vi "OCT with Classes - ATS6350.vi"() -> ()   [LabVIEW 2014]
doc: "I. Description:\nThis example demonstrates how to acquire a continuous amount of data (Waveform) using the DAQ device's internal clock.\n\nII. Instructions for Running:\n1. Create an analog input voltage channel.\n2. Set the rate for the sample clock. Additionally, define the sample mode to be continuous.\n3. Call the Start VI to start the acquisition.\n4. Read the waveform data in a loop until the user hits the stop button or an error occurs.\nNote: This example reads data from one or more channels and returns an array of data. Use the Index Array function to access an individual channel of data.\n5. Call the Clear Task VI to clear the Task.\n6. Use the popup dialog box to display an error if any.\n\nIV. I/O Connections Overview:\nMake sure your signal input terminal matches the Physical Channel I/O Control. For further connection information, refer to your hardware reference manual."
uses:
  Type Defs/OCT DAQ Channel Data Type.ctl
  Type Defs/OCT Hardware States.ctl
  Classes/Galvo/Scanning Cluster.ctl
  Classes/Galvo/NI Galvo/NI Galvo.lvclass
  Processing Class/Intensity/Intensity Processing.lvclass
  Classes/DAQ/ATS9350/ATS9350.lvclass
  Classes/DAQ/DAQ Parameters.ctl
  Classes/DAQ/Trigger Source.ctl
  Classes/DAQ/Trigger Slope.ctl
  Classes/DAQ/Clock Control.ctl
  Classes/Laser/Insite/Insight.lvclass
  Classes/DAQ Control Functional Global States.ctl
  DAQ Status States.ctl
  Signal Processing/processing_states.ctl
  Signal Processing/Display Raw Data states.ctl
  Classes/Processing/View A-Scan.vi
  Classes/DAQ/DAQ Class.lvclass
  Classes/Processing.lvclass
  Classes/Galvo/Galvo.lvclass
panel:
  in  "Laser Status":string
  out "Single A-Scan":u16[](graph)
  in  "Scanning Parameters":T1={"Fast Axis Offset"=0.0, "Slow Axis Offset"=0.0, "Slow Axis Amp"=2.0, "Fast Axis Amp"=2.0, "Scan Pattern"=enum."Raster"} {"Fast Axis Amp" max=20 format="%#.2f"; "Slow Axis Amp" max=20 format="%#.2f"; "Slow Axis Offset" max=10 format="%#.2f"; "Fast Axis Offset" max=10 format="%#.2f"}
  out "Log10?":bool
  in  "OCT Hardware States":T2
  out "Background Array":u16[](array[numeric])
  in  "Calibrate":bool
  in  "Save Sweep Button":bool
  in  "Data Format":T3
  in  "Save Sweep":bool
  in  "Stop Button":bool
  out "B-Scans Per Buffer":i32=1
  out "Clock Length":u32=9184
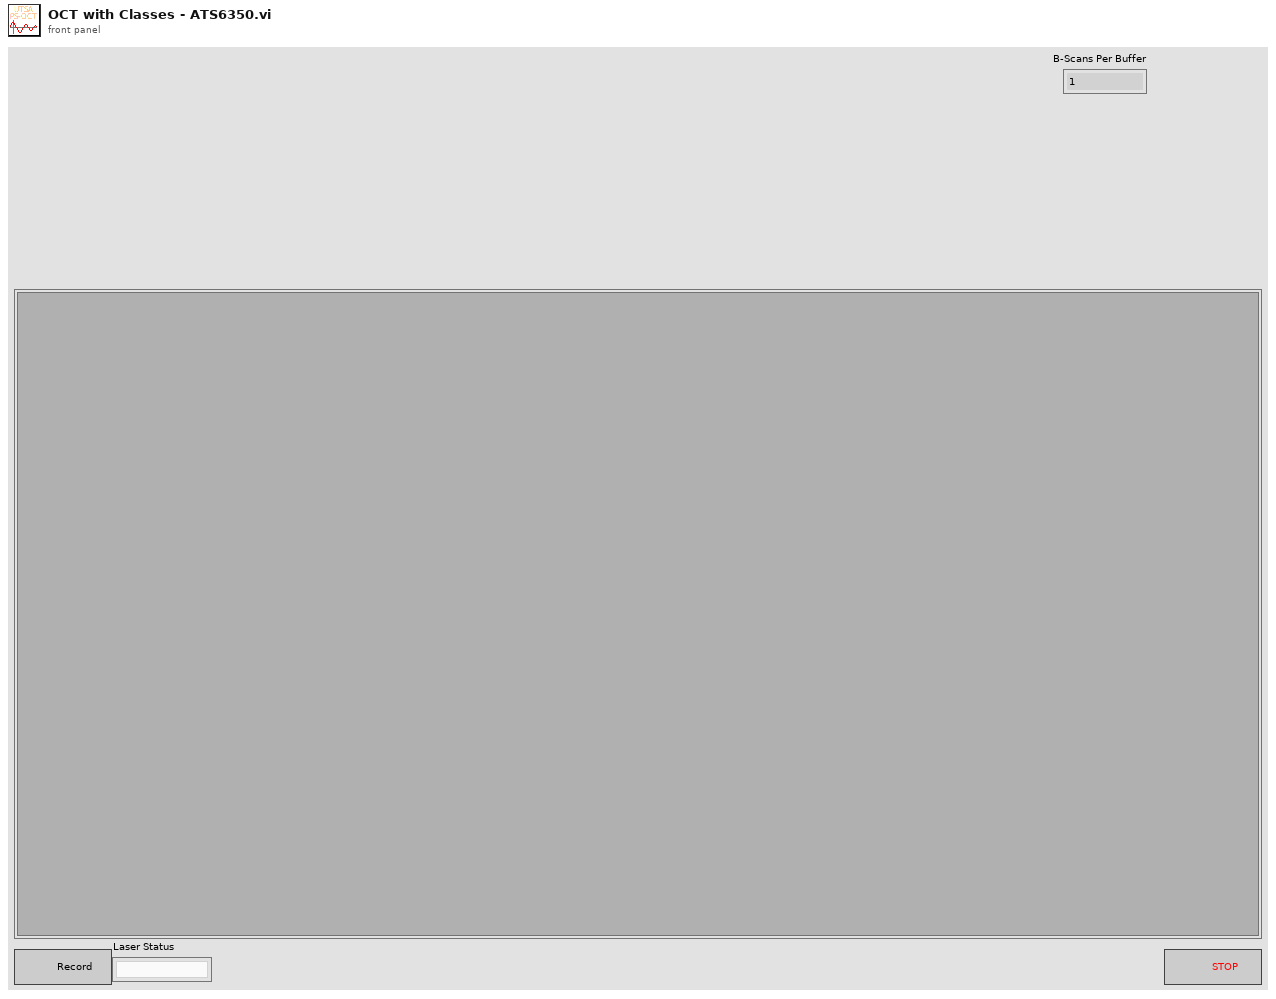
[diagram p1: front panel]
types:
  T1 = typedef "Galvo.lvclass/Scanning Cluster.ctl" = cluster{"Fast Axis Offset":sgl, "Slow Axis Offset":sgl, "Slow Axis Amp":sgl, "Fast Axis Amp":sgl, "Scan Pattern":enum16{"Raster"}}
  T2 = typedef "OCT Hardware States.ctl" = enum16{"Acquire Data", "Initialize Laser", "Initialize Galvos", "Startup", "Reset DAQ", "Background Subtraction", "Acquire Background", "Update DAQ Parameters", "Stop", "Set Clock", "Initialize DAQ", "Set Resampling Array", "Save Sweep", "Configure Laser"}
  T3 = typedef "OCT DAQ Channel Data Type.ctl" = enum16{"Channel 1", "Channel 2", "Channel 1 and 2"}
  T4 = typedef "DAQ Class.lvclass/DAQ Parameters.ctl" = cluster{"Points Per A-Scan":u32, "A-Scans Per B-Scan":u32, "Number of B-Scans":u32, "A-Scans Per Transfer":u32, "Trigger Voltage":sgl, "Trigger Source":T5, "Trigger Slope":T6, "Channel":T3, "Clock":T7, "Bits per Sample":dbl, "Range":dbl}
  T5 = typedef "DAQ Class.lvclass/Trigger Source.ctl" = enum16{"External", "Channel A", "Channel B"}
  T6 = typedef "DAQ Class.lvclass/Trigger Slope.ctl" = enum16{"Rising", "Falling"}
  T7 = typedef "DAQ Class.lvclass/Clock Control.ctl" = enum16{"Internal Clock", "External Clock"}
  T8 = typedef "DAQ Control Functional Global States.ctl" = enum16{"Status", "Set Processing Finished", "Reset", "Clear", "Set DAQ Finished"}
  T9 = enum32{"Invalid", "Standard", "Closed", "Hidden", "Minimized", "Maximized"}
  T10 = typedef "DAQ Status States.ctl" = enum16{"Get", "Show"}
  T11 = typedef "Display Raw Data states.ctl" = enum16{"Add Raw", "Add Processed", "Show"}
  T12 = typedef "processing_states.ctl" = enum16{"Initialize", "Set Background", "Update Imaging Parameters", "Get Queue", "Process Data", "Get Size", "Flush Data", "Set Reample Array", "Get Last Processed BScan", "Shutdown"}
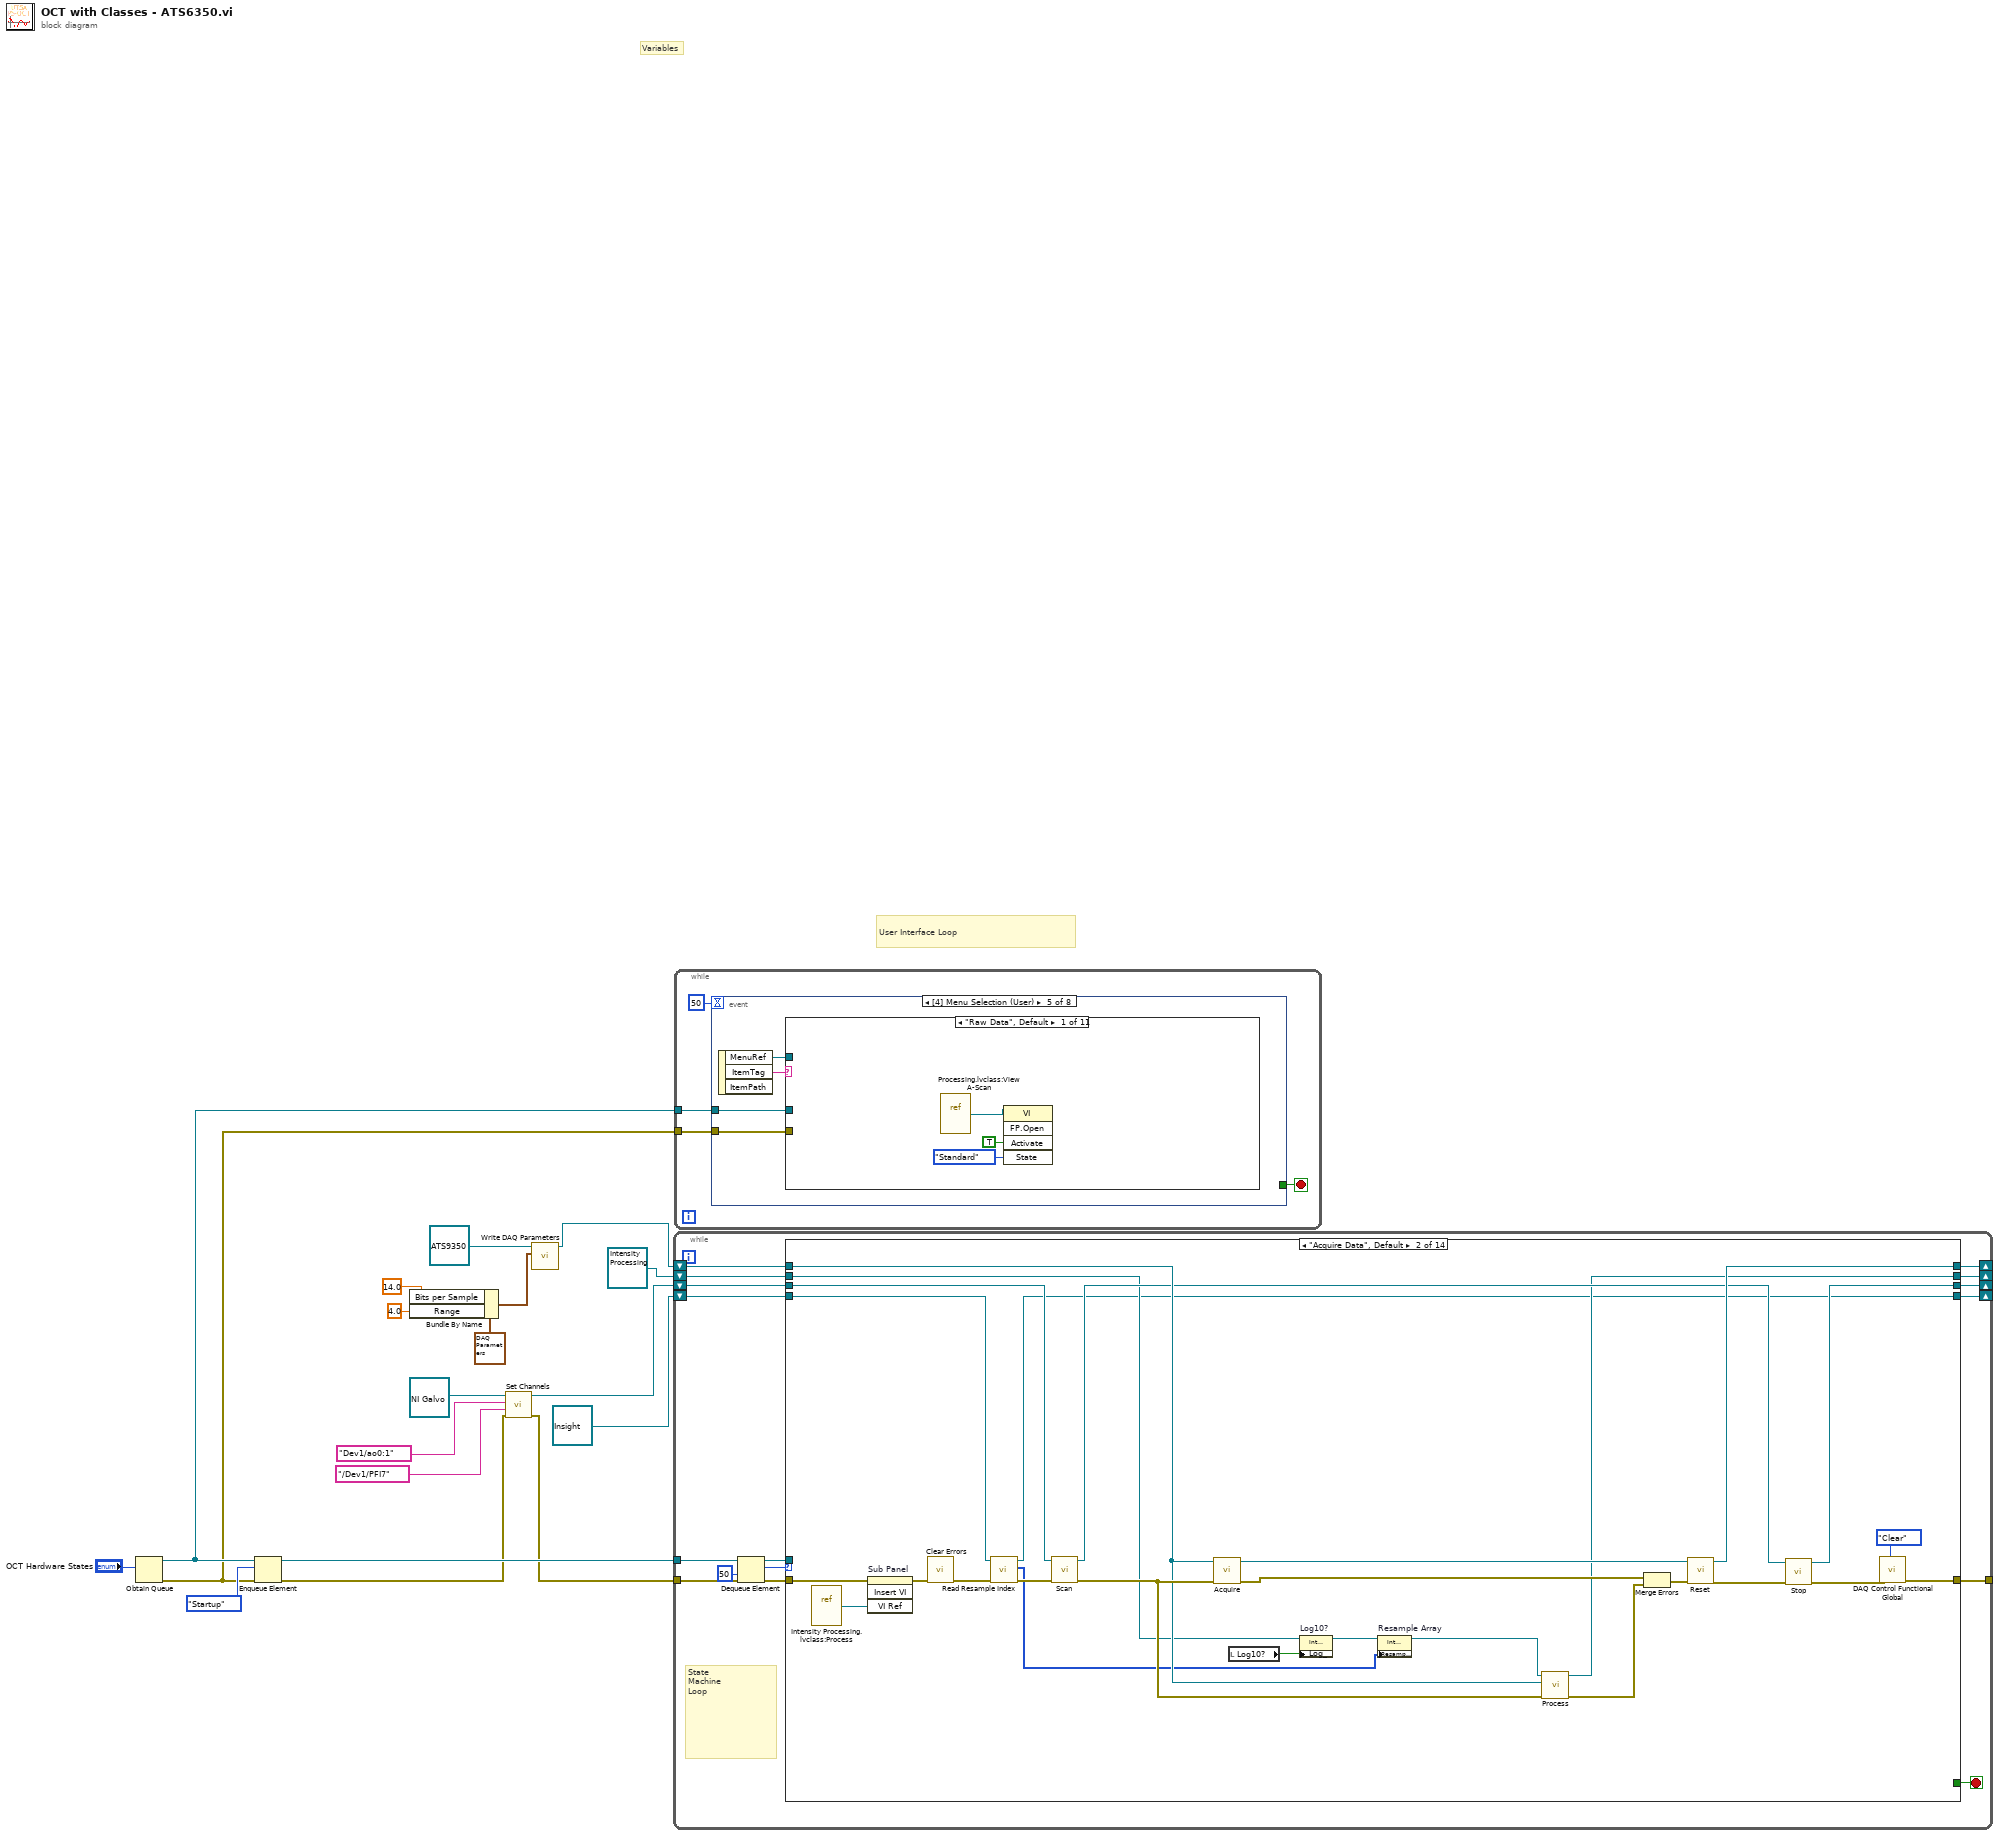
[diagram p0: block diagram]
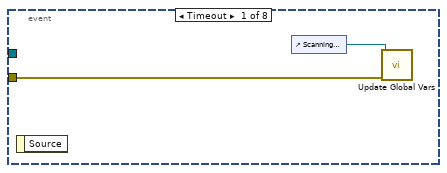
[diagram p2: hidden frame]
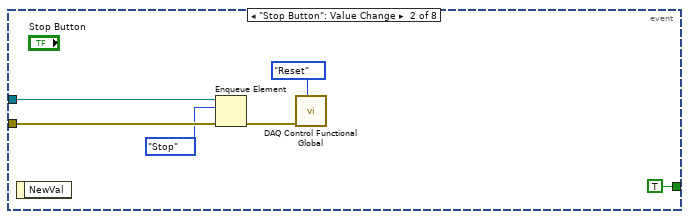
[diagram p3: hidden frame]
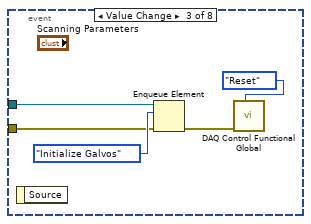
[diagram p4: hidden frame]
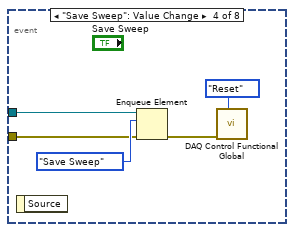
[diagram p5: hidden frame]
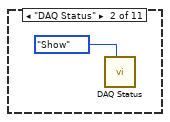
[diagram p6: hidden frame]
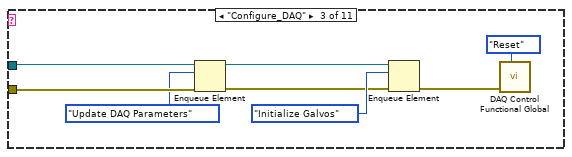
[diagram p7: hidden frame]
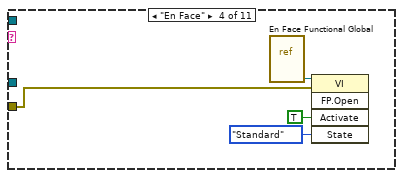
[diagram p8: hidden frame]
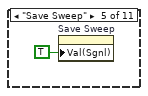
[diagram p9: hidden frame]
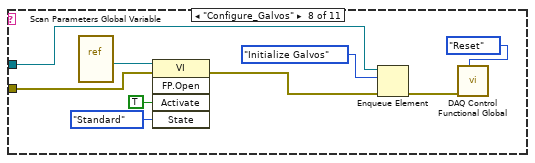
[diagram p12: hidden frame]
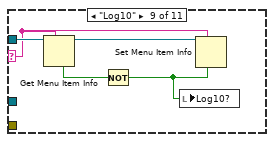
[diagram p13: hidden frame]
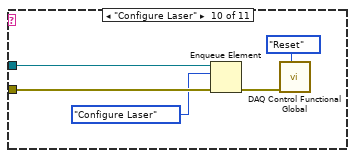
[diagram p14: hidden frame]
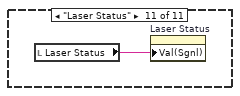
[diagram p15: hidden frame]
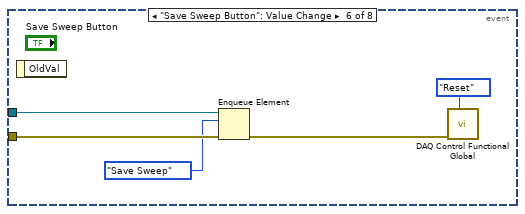
[diagram p16: hidden frame]
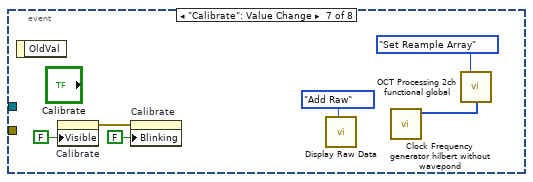
[diagram p17: hidden frame]
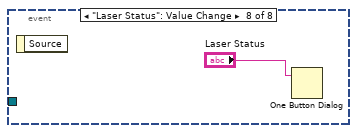
[diagram p18: hidden frame]
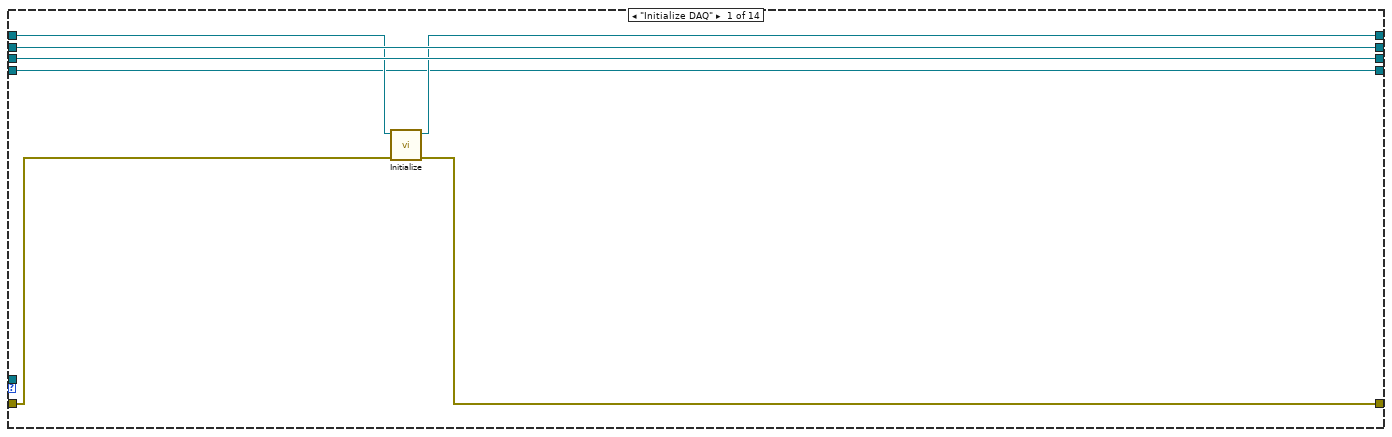
[diagram p19: hidden frame]
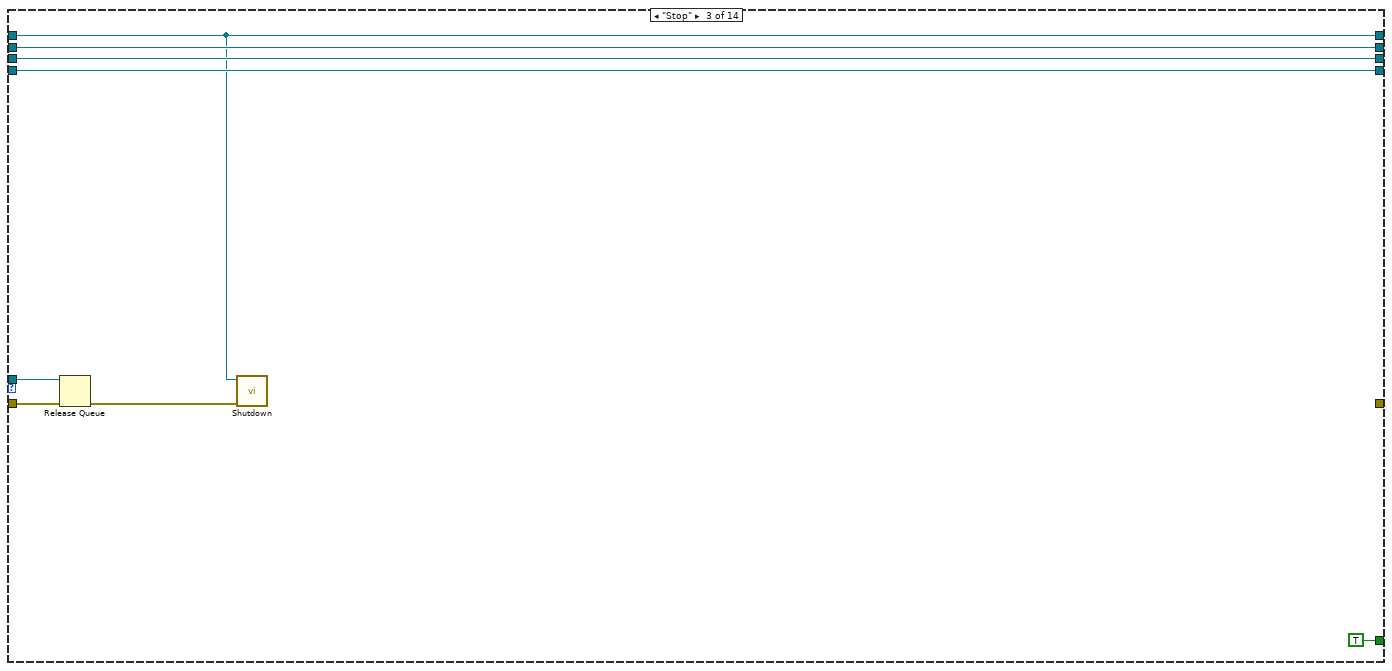
[diagram p20: hidden frame]
diagram:
  # "User Interface Loop"
  # "Variables"
  n1 = Obtain Queue(element data type="OCT Hardware States") -> (queue out=w17:refnum<queue>, error out=w15:errorcluster)  [unwired: 4 in, 1 out]
  n2 = Enqueue Element(queue=w17, element=OCT_Hardware_States."Startup", error in (no error)=w15) -> (queue out=w18:refnum<queue>, error out=w6:errorcluster)  [unwired: 1 in, 1 out]
  n3 = Bundle By Name(cluster=T4 {"Points Per A-Scan"=1024, "A-Scans Per B-Scan"=250, "Number of B-Scans"=1, "A-Scans Per Transfer"=1, "Trigger Voltage"=140.0, "Trigger Source"=enum."External", "Trigger Slope"=enum."Rising", "Channel"=enum."Channel 1", "Clock"=enum."Internal Clock", "Bits per Sample"=16.0, "Range"=4.0} ("DAQ Parameters"), "Bits per Sample"=14.0, "Range"=4.0) -> (w10:T4)
  n4 = call-dynamic "Set Channels.vi"("error in (no error)"=w6, "Trigger Source"=tag "/Dev1/PFI7", "Analog Output"=tag "Dev1/ao0:1", "NI Galvo in"=refnum<class "NI Galvo.lvclass"> refnum ("NI Galvo.lvclass")) -> ("error out"=w5:errorcluster, "NI Galvo out"=w4:refnum<class "NI Galvo.lvclass">)  [unwired: 6 in]
  n5 = call-dynamic "Write DAQ Parameters.vi"("DAQ Parameters"=w10, "ATS9350 in"=refnum<class "ATS9350.lvclass"> refnum ("ATS9350.lvclass")) -> ("ATS9350 out"=w12:refnum<class "ATS9350.lvclass">)  [unwired: 8 in, 1 out]
  n6 = while {
    tunnel: w18 -> [w35]
    tunnel: w5 -> [w30]
    tunnel: [w31] -> _
    shift-right: [w27] -> _
    shift-left: w12 -> [w28]
    shift-right: [w23] -> _
    shift-left: refnum<class "Intensity Processing.lvclass"> refnum ("Intensity Processing.lvclass") -> [w26]
    shift-right: [w22] -> _
    shift-left: w4 -> [w25]
    shift-right: [w21] -> _
    shift-left: refnum<class "Insight.lvclass"> refnum ("Insight.lvclass") -> [w24]
    stop <- w20 stop-if-true
    # "State\nMachine\nLoop"
    n7 = Dequeue Element(queue=w35, timeout in ms (-1)=50, error in (no error)=w30) -> (queue out=w33:refnum<queue>, element=w29:T2, error out=w34:errorcluster)  [unwired: 1 out]
    n8 = case shown="\"Acquire Data\", Default" w29 {
      tunnel: w34 -> [w37 w59 w76 w87 _ _ w115 _ w126 w157 w165 _ w179 w189]
      tunnel: w33 -> [_ _ w77 _ _ _ _ _ w127 w156 _ _ _ _]
      tunnel: [w42 w68 _ w78 _ _ w97 _ _ w154 w168 _ w177 w184] -> w31
      tunnel: w28 -> [w39 w56 w71 w80 w91 w95 w105 w122 w132 w153 w160 w175 w182 w192]
      tunnel: [w38 w55 w71 w79 w91 w95 w98 w122 w132 w152 w159 w175 w182 w192] -> w27
      tunnel: w26 -> [w41 w52 w74 w83 w90 w94 w107 w121 w131 w151 w164 w174 w181 w191]
      tunnel: w25 -> [w40 w57 w73 w82 w89 w93 w106 w120 w130 w150 w162 w173 w180 w190]
      tunnel: w24 -> [w36 w47 w72 w81 w88 w92 w96 w119 w129 w149 w163 w172 w178 w186]
      tunnel: [w41 w51 w74 w83 w90 w94 w107 w121 w131 w151 w164 w174 w181 w191] -> w23
      tunnel: [w40 w53 w73 w82 w89 w93 w106 w120 w130 w150 w161 w173 w180 w190] -> w22
      tunnel: [w36 w46 w72 w81 w88 w92 w96 w119 w129 w149 w163 w172 w176 w185] -> w21
      tunnel: [_ _ TRUE _ _ _ _ _ _ _ _ _ _ _] -> w20
      frame "Initialize DAQ" {
        n9 = call-dynamic "Initialize.vi"("error in (no error)"=w37, "ATS9350 in"=w39) -> ("error out"=w42:errorcluster, "ATS9350 out"=w38:refnum<class "ATS9350.lvclass">)  [unwired: 8 in]
      }
      frame "Acquire Data", Default {
        n10 = vi-ref "Intensity Processing.lvclass:Process.vi"() -> (w58:refnum<vi>)
        n11 = invoke on="Sub Panel" class="SubPanel" method="Insert VI"(error in=w59, "VI Ref"=w58) -> (error out=w50:errorcluster)  [unwired: 2 in, 3 out]
        n12 = call <vilib>:"Clear Errors.vi"("error in (no error)"=w50) -> ("error out"=w49:errorcluster)  [unwired: 5 in, 1 out]
        n13 = call-dynamic "Read Resample Index.vi"("error in (no error)"=w49, "Laser in"=w47) -> ("error out"=w48:errorcluster, "Resample Index"=w44:u32[], "Laser out"=w46:refnum<class "Insight.lvclass">)  [unwired: 7 in]
        n14 = call-dynamic "Scan.vi"("error in (no error)"=w48, "NI Galvo in"=w57) -> ("error out"=w62:errorcluster, "NI Galvo out"=w54:refnum<class "NI Galvo.lvclass">)  [unwired: 8 in]
        n15 = call-dynamic "Acquire.vi"("error in (no error)"=w62, "ATS9350 in"=w56) -> ("error out"=w66:errorcluster, "ATS9350 out"=w64:refnum<class "ATS9350.lvclass">)  [unwired: 8 in]
        n16 = local read "Log10?"() -> (w63:bool)
        n17 = property on="Log10?" class="Intensity Processing.lvclass"(reference=w52, "Log_"=w63) -> (reference out=w45:refnum<class "Intensity Processing.lvclass">)  [unwired: 1 in, 1 out]
        n18 = property on="Resample Array" class="Intensity Processing.lvclass"(reference=w45, "Resample Array"=w44) -> (reference out=w43:refnum<class "Intensity Processing.lvclass">)  [unwired: 1 in, 1 out]
        n19 = call-dynamic "Process.vi"("error in (no error)"=w62, "DAQ Class.lvclass"=w56, "Intensity Processing in"=w43) -> ("error out"=w67:errorcluster, "Intensity Processing out"=w51:refnum<class "Intensity Processing.lvclass">)  [unwired: 7 in]
        n20 = Merge Errors(w66, w67) -> (w65:errorcluster)
        n21 = call-dynamic "Reset.vi"("error in (no error)"=w65, "ATS9350 in"=w64) -> ("error out"=w61:errorcluster, "ATS9350 out"=w55:refnum<class "ATS9350.lvclass">)  [unwired: 8 in]
        n22 = call-dynamic "Stop.vi"("error in (no error)"=w61, "NI Galvo in"=w54) -> ("error out"=w60:errorcluster, "NI Galvo out"=w53:refnum<class "NI Galvo.lvclass">)  [unwired: 8 in]
        n23 = call "DAQ Control Functional Global.vi"("State"=DAQ_Control_Functional_Global_States."Clear", "Error In"=w60) -> ("Error Out"=w68:errorcluster)  [unwired: 6 in, 3 out]
      }
      frame "Stop" {
        n24 = Release Queue(queue=w77, error in (no error)=w76) -> (error out=w75:errorcluster)  [unwired: 1 in, 2 out]
        n25 = call-dynamic "Shutdown.vi"("error in (no error)"=w75, "ATS9350 in"=w71) -> ()  [unwired: 8 in, 2 out]
      }
      frame "Update DAQ Parameters" {
        n26 = call-dynamic "Update DAQ Parameters.vi"("error in (no error)"=w87, "DAQ Class in"=w80) -> ("error out"=w85:errorcluster, "DAQ Parameters Out"=w84:T4, "DAQ Class out"=w86:refnum<class "ATS9350.lvclass">)  [unwired: 7 in]
        n27 = call-dynamic "Write DAQ Parameters.vi"("error in (no error)"=w85, "DAQ Parameters"=w84, "ATS9350 in"=w86) -> ("error out"=w78:errorcluster, "ATS9350 out"=w79:refnum<class "ATS9350.lvclass">)  [unwired: 7 in]
      }
      frame "Background Subtraction" {
      }
      frame "Acquire Background" {
      }
      frame "Set Clock" {
        n28 = call "DAQ Control Functional Global.vi"("State"=DAQ_Control_Functional_Global_States."Clear", "Error In"=w115) -> ("Error Out"=w114:errorcluster)  [unwired: 6 in, 3 out]
        n29 = call "Compute 1 A-Scan Parameters.vi"("error in (no error)"=w114, "Laser In"=w96, "ATS660 Class.lvclass in"=w105) -> ("error out"=w108:errorcluster, "DAQ Parameters"=w104:T4, "ATS660 Class out"=w109:refnum<class "ATS9350.lvclass">)  [unwired: 6 in]
        n30 = Bundle By Name(cluster=w104, "Trigger Voltage"=sgl 140.0) -> (w102:T4)
        n31 = call-dynamic "Write DAQ Parameters.vi"("error in (no error)"=w108, "DAQ Parameters"=w102, "ATS9350 in"=w109) -> ("error out"=w113:errorcluster, "ATS9350 out"=w112:refnum<class "ATS9350.lvclass">)  [unwired: 7 in]
        n32 = call-dynamic "Reset.vi"("error in (no error)"=w113, "ATS9350 in"=w112) -> ("error out"=w110:errorcluster, "ATS9350 out"=w111:refnum<class "ATS9350.lvclass">)  [unwired: 8 in]
        n33 = call-dynamic "Acquire.vi"("error in (no error)"=w110, "ATS9350 in"=w111) -> ("error out"=w117:errorcluster, "ATS9350 out"=w118:refnum<class "ATS9350.lvclass">)  [unwired: 8 in]
        n34 = call-dynamic "Get Last Buffer.vi"("error in (no error)"=w117, "DAQ Class in"=w118) -> ("error out"=w100:errorcluster, "Last Buffer"=→"Single A-Scan":u16[], "DAQ Class out"=w99:refnum<class "ATS9350.lvclass">)  [unwired: 7 in]
        n35 = call-dynamic "Reset.vi"("error in (no error)"=w100, "ATS9350 in"=w99) -> ("error out"=w97:errorcluster, "ATS9350 out"=w98:refnum<class "ATS9350.lvclass">)  [unwired: 8 in]
        n36 = call "Clock Frequency generator hilbert.vi"() -> ()  [unwired: 10 in, 2 out]
      }
      frame "Set Resampling Array" {
      }
      frame "Startup" {
        n37 = Enqueue Element(queue=w127, element=OCT_Hardware_States."Initialize Laser", error in (no error)=w126) -> (queue out=w124:refnum<queue>, error out=w125:errorcluster)  [unwired: 1 in, 1 out]
        n38 = Enqueue Element(queue=w124, element=OCT_Hardware_States."Initialize DAQ", error in (no error)=w125) -> (queue out=w136:refnum<queue>, error out=w135:errorcluster)  [unwired: 1 in, 1 out]
        n39 = Enqueue Element(queue=w136, element=OCT_Hardware_States."Set Clock", error in (no error)=w135) -> (queue out=w134:refnum<queue>, error out=w133:errorcluster)  [unwired: 1 in, 1 out]
        n40 = local write "Stop Button"(FALSE ("Sweep Ready for saving")) -> ()
        n41 = Enqueue Element(queue=w134, element=OCT_Hardware_States."Update DAQ Parameters", error in (no error)=w133) -> (queue out=w146:refnum<queue>, error out=w145:errorcluster)  [unwired: 1 in, 1 out]
        n42 = Enqueue Element(queue=w146, element=OCT_Hardware_States."Initialize Galvos", error in (no error)=w145) -> (queue out=w139:refnum<queue>, error out=w138:errorcluster)  [unwired: 1 in, 1 out]
        n43 = Enqueue Element(queue=w139, element=OCT_Hardware_States."Acquire Data", error in (no error)=w138) -> ()  [unwired: 1 in, 3 out]
        "B-Scans Per Buffer" <- 4 ("B-Scans Per Buffer")
        "Clock Length" <- u32 9184 ("Clock Length")
        "Log10?" <- TRUE ("Log10?")
      }
      frame "Save Sweep" {
        n44 = Enqueue Element(queue=w156, element=OCT_Hardware_States."Acquire Data", error in (no error)=w157) -> (error out=w155:errorcluster)  [unwired: 1 in, 2 out]
        n45 = call-dynamic "Save.vi"("error in (no error)"=w155, "DAQ Class in"=w153) -> ("error out"=w154:errorcluster, "DAQ Class out"=w152:refnum<class "ATS9350.lvclass">)  [unwired: 8 in]
      }
      frame "Initialize Galvos" {
        n46 = call-dynamic "Read DAQ Parameters.vi"("error in (no error)"=w165, "ATS9350 in"=w160) -> ("error out"=w166:errorcluster, "DAQ Parameters"=w167:T4, "ATS9350 out"=w159:refnum<class "ATS9350.lvclass">)  [unwired: 7 in]
        n47 = local read "Scanning Parameters"() -> (w171:T1)
        n48 = call-dynamic "Configure.vi"("error in (no error)"=w166, "DAQ Parameters"=w167, "Scanning Parameters"=w171, "NI Galvo in"=w162) -> ("error out"=w170:errorcluster, "NI Galvo out"=w169:refnum<class "NI Galvo.lvclass">)  [unwired: 6 in]
        n49 = call-dynamic "Initialize.vi"("error in (no error)"=w170, "NI Galvo in"=w169) -> ("error out"=w168:errorcluster, "NI Galvo out"=w161:refnum<class "NI Galvo.lvclass">)  [unwired: 8 in]
      }
      frame "Reset DAQ" {
      }
      frame "Configure Laser" {
        n50 = call-dynamic "Configure.vi"("error in (no error)"=w179, "Insight in"=w178) -> ("error out"=w177:errorcluster, "Insight out"=w176:refnum<class "Insight.lvclass">)  [unwired: 8 in]
      }
      frame "Initialize Laser" {
        n51 = call-dynamic "Init.vi"("error in (no error)"=w189, "Insite in"=w186) -> ("error out"=w187:errorcluster, "Insite out"=w188:refnum<class "Insight.lvclass">)  [unwired: 8 in]
        n52 = call-dynamic "Read Status.vi"("error in (no error)"=w187, "Laser in"=w188) -> ("error out"=w184:errorcluster, "Status"=w183:string, "Laser out"=w185:refnum<class "Insight.lvclass">)  [unwired: 7 in]
        n53 = local write "Laser Status"(w183) -> ()
      }
    }
  }
  n54 = while {
    tunnel: w17 -> [w196]
    tunnel: w15 -> [w195]
    stop <- w193 stop-if-true
    n55 = event shown="[4] Menu Selection (User)" {
      selector: _ -> [_ _ _ _ _ _ _ _]
      dyn-events: _ -> [_ _ _ _ _ _ _ _]
      timeout: 50 -> [_ _ _ _ _ _ _ _]
      tunnel: w196 -> [_ w203 w206 w211 w217 w257 _ _]
      tunnel: w195 -> [w197 w204 w207 w212 w216 w259 _ _]
      tunnel: [_ TRUE _ _ _ _ _ _] -> w193
      event Timeout {
        n56 = event-data() -> ()  [unwired: 1 in, 1 out]
        n57 = control-ref of="Scanning Parameters"() -> (w198:refnum<vi>)
        n58 = call "Update Global Vars.vi"("Error In"=w197, "Cluster in"=w198) -> ()  [unwired: 9 in, 1 out]
      }
      event "Stop Button": Value Change {
        n59 = event-data() -> ()  [unwired: 1 in, 1 out]
        n60 = Enqueue Element(queue=w203, element=OCT_Hardware_States."Stop", error in (no error)=w204) -> (error out=w201:errorcluster)  [unwired: 1 in, 2 out]
        n61 = call "DAQ Control Functional Global.vi"("State"=DAQ_Control_Functional_Global_States."Reset", "Error In"=w201) -> ()  [unwired: 6 in, 4 out]
      }
      event Value Change {
        n62 = event-data() -> ()  [unwired: 1 in, 1 out]
        n63 = Enqueue Element(queue=w206, element=OCT_Hardware_States."Initialize Galvos", error in (no error)=w207) -> (error out=w208:errorcluster)  [unwired: 1 in, 2 out]
        n64 = call "DAQ Control Functional Global.vi"("State"=DAQ_Control_Functional_Global_States."Reset", "Error In"=w208) -> ()  [unwired: 6 in, 4 out]
      }
      event "Save Sweep": Value Change {
        n65 = event-data() -> ()  [unwired: 1 in, 1 out]
        n66 = Enqueue Element(queue=w211, element=OCT_Hardware_States."Save Sweep", error in (no error)=w212) -> (error out=w210:errorcluster)  [unwired: 1 in, 2 out]
        n67 = call "DAQ Control Functional Global.vi"("State"=DAQ_Control_Functional_Global_States."Reset", "Error In"=w210) -> ()  [unwired: 6 in, 4 out]
      }
      event Menu Selection (User) {
        n68 = event-data() -> ("MenuRef"=w215:refnum<k9>, "ItemTag"=w218:string)  [unwired: 1 in, 1 out]
        n69 = case shown="\"Raw Data\", Default" w218 {
          selector: w218 -> [_ _ _ _ _ _ _ _ w246 _ _]
          tunnel: w217 -> [_ _ w230 _ _ _ _ w238 _ w254 _]
          tunnel: w216 -> [_ _ w229 w231 _ _ _ w236 _ w253 _]
          tunnel: w215 -> [_ _ _ _ _ _ _ _ w249 _ _]
          frame "Raw Data", Default {
            n70 = vi-ref "Processing.lvclass:View A-Scan.vi"() -> (w221:refnum<vi>)
            n71 = invoke class="VI" method="FP.Open"(reference=w221, "Activate"=TRUE ("Activate?"), "State"=T9."Standard") -> ()  [unwired: 2 in, 5 out]
          }
          frame "DAQ Status" {
            n72 = call "DAQ Status.vi"("Enum"=DAQ_Status_States."Show") -> ()  [unwired: 9 in, 2 out]
          }
          frame "Configure_DAQ" {
            n73 = Enqueue Element(queue=w230, element=OCT_Hardware_States."Update DAQ Parameters", error in (no error)=w229) -> (queue out=w224:refnum<queue>, error out=w225:errorcluster)  [unwired: 1 in, 1 out]
            n74 = Enqueue Element(queue=w224, element=OCT_Hardware_States."Initialize Galvos", error in (no error)=w225) -> (error out=w223:errorcluster)  [unwired: 1 in, 2 out]
            n75 = call "DAQ Control Functional Global.vi"("State"=DAQ_Control_Functional_Global_States."Reset", "Error In"=w223) -> ()  [unwired: 6 in, 4 out]
          }
          frame "En Face" {
            n76 = vi-ref "En Face Functional Global.vi"() -> (w232:refnum<vi>)
            n77 = invoke class="VI" method="FP.Open"(reference=w232, error in=w231, "Activate"=TRUE ("Activate?"), "State"=T9."Standard") -> ()  [unwired: 1 in, 5 out]
          }
          frame "Save Sweep" {
            n78 = property on="Save Sweep" class="Bool (strict)"("Val(Sgnl)"=TRUE ("Value (Signaling)")) -> ()  [unwired: 2 in, 2 out]
          }
          frame "K-Space Correction" {
          }
          frame "Background Subtraction" {
          }
          frame "Configure_Galvos" {
            n79 = vi-ref "Scan Parameters Global Variable.vi"() -> (w244:refnum<vi>)
            n80 = invoke class="VI" method="FP.Open"(reference=w244, error in=w236, "Activate"=TRUE ("Activate?"), "State"=T9."Standard") -> (error out=w237:errorcluster)  [unwired: 1 in, 4 out]
            n81 = Enqueue Element(queue=w238, element=OCT_Hardware_States."Initialize Galvos", error in (no error)=w237) -> (error out=w240:errorcluster)  [unwired: 1 in, 2 out]
            n82 = call "DAQ Control Functional Global.vi"("State"=DAQ_Control_Functional_Global_States."Reset", "Error In"=w240) -> ()  [unwired: 6 in, 4 out]
          }
          frame "Log10" {
            n83 = Get Menu Item Info(7:w246, 11:w249) -> (3:w247:refnum<k9>, 4:w248:bool)  [unwired: 1 in, 5 out]
            n84 = Not(x=w248) -> (.not. x?=w245:bool)
            n85 = local write "Log10?"(w245) -> ()
            n86 = Set Menu Item Info(6:w245, 7:w246, 11:w247) -> ()  [unwired: 4 in, 2 out]
          }
          frame "Configure Laser" {
            n87 = Enqueue Element(queue=w254, element=OCT_Hardware_States."Configure Laser", error in (no error)=w253) -> (error out=w250:errorcluster)  [unwired: 1 in, 2 out]
            n88 = call "DAQ Control Functional Global.vi"("State"=DAQ_Control_Functional_Global_States."Reset", "Error In"=w250) -> ()  [unwired: 6 in, 4 out]
          }
          frame "Laser Status" {
            n89 = local read "Laser Status"() -> (w255:string)
            n90 = property on="Laser Status" class="Str"("Val(Sgnl)"=w255) -> ()  [unwired: 2 in, 2 out]
          }
        }
      }
      event "Save Sweep Button": Value Change {
        n91 = event-data() -> ()  [unwired: 1 in, 1 out]
        n92 = Enqueue Element(queue=w257, element=OCT_Hardware_States."Save Sweep", error in (no error)=w259) -> (error out=w258:errorcluster)  [unwired: 1 in, 2 out]
        n93 = call "DAQ Control Functional Global.vi"("State"=DAQ_Control_Functional_Global_States."Reset", "Error In"=w258) -> ()  [unwired: 6 in, 4 out]
      }
      event "Calibrate": Value Change {
        n94 = event-data() -> ()  [unwired: 1 in, 1 out]
        n95 = property on="Calibrate" class="Bool"("Visible"=FALSE) -> (error out=w265:errorcluster)  [unwired: 2 in, 1 out]
        n96 = property on="Calibrate" class="Bool"(error in=w265, "Blinking"=FALSE) -> ()  [unwired: 1 in, 2 out]
        n97 = call "Display Raw Data.vi"("Enum"=Display_Raw_Data_states."Add Raw") -> ()  [unwired: 11 in]
        n98 = call "Clock Frequency generator hilbert without wavepond.vi"() -> ("Zero Crossing Resample Index"=w261:i32[])  [unwired: 11 in]
        n99 = call "OCT Processing 2ch functional global.vi"("State"=processing_states."Set Reample Array", "Resample Array"=w261) -> ()  [unwired: 9 in, 5 out]
      }
      event "Laser Status": Value Change {
        n100 = event-data() -> ()  [unwired: 1 in, 1 out]
        n101 = One Button Dialog(message="Laser Status") -> ()  [unwired: 1 in, 1 out]
      }
    }
  }
